vi "single cycle kalman step.vi"(0 "state in":T1, 1 "apply measurement":bool, 2 "z-offset":i16, 5 "location":T4, 9 "pixel values cluster":T3, 11 "feedback channel":enum16{"channel 0", "channel 1", "both"}(ring)=enum."both", 13 "Vz feedback?":bool, 14 "Vxy feedback":bool=TRUE) -> (4 "state out":T1, 8 "kalman counting":bool)   [LabVIEW 2010]
uses:
  kalman 3-axis state.ctl
  integrating single axis kalman state.ctl
  common_typedefs/channels_cluster.ctl
panel:
  # "1 z-level = 3.4*10^-4 * scan amplitude\nat A = 30 um, 1 z-level = 10 nm"
  # "full scan range -> half valid z > 9143 (=143 * 64)"
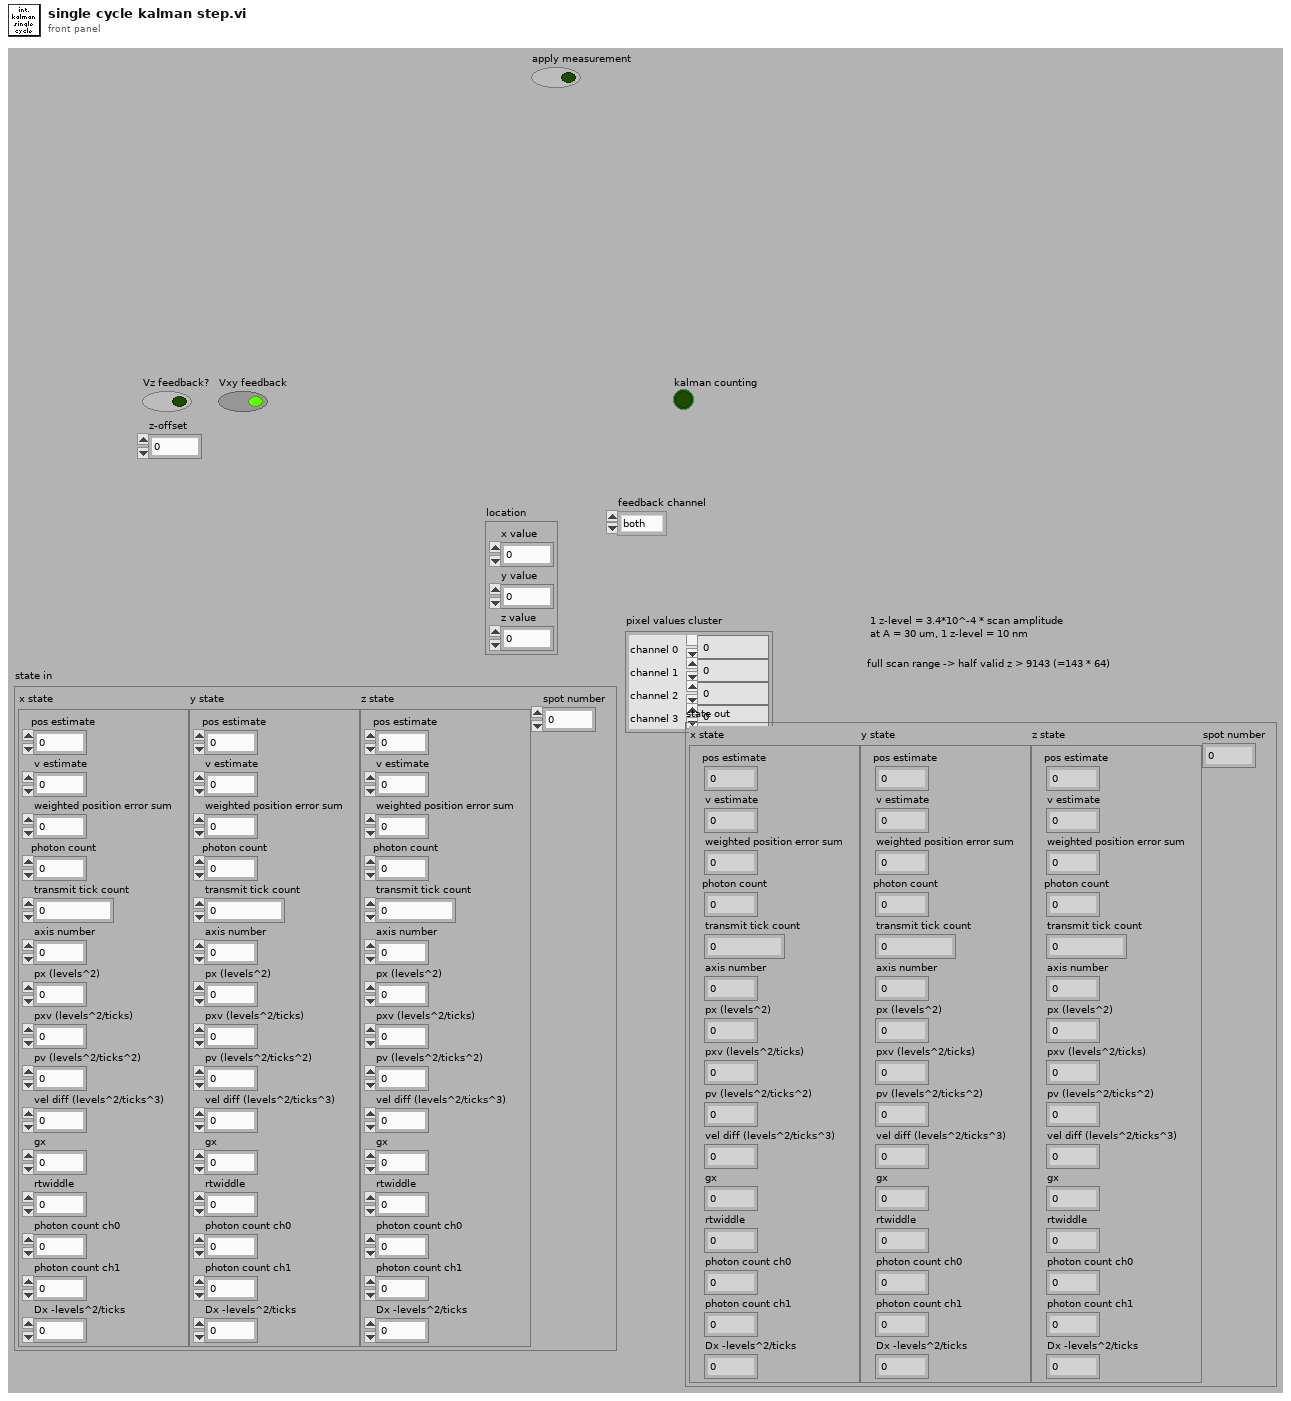
[diagram p1: front panel]
types:
  T1 = typedef "kalman 3-axis state.ctl" = cluster{"x state":T2, "y state":T2, "z state":T2, "spot number":u8}
  T2 = typedef "integrating single axis kalman state.ctl" = cluster{"pos estimate":fxp<+/-,32,16>, "v estimate":fxp<+/-,16,0>, "weighted position error sum":fxp<+/-,32,32>, "photon count":u32, "transmit tick count":u32, "axis number":u8, "px (levels^2)":fxp<+,32,19>, "pxv (levels^2/ticks)":fxp<+,32,2>, "pv (levels^2/ticks^2)":fxp<+,32,-14>, "vel diff (levels^2/ticks^3)":fxp<+,24,-22>, "gx":fxp<+,16,8>, "rtwiddle":fxp<+,16,26>, "photon count ch0":u32, "photon count ch1":u32, "Dx -levels^2/ticks":fxp<+,32,19>}
  T3 = typedef "channels_cluster.ctl" = cluster{"channel 0":u32, "channel 1":u32, "channel 2":u32, "channel 3":u32}
  T4 = cluster{"x value":i16, "y value":i16, "z value":i16}
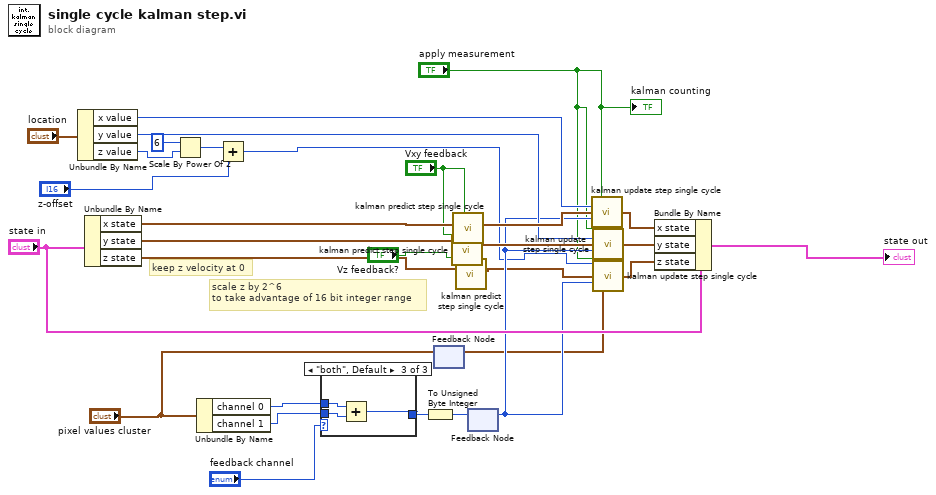
[diagram p0: block diagram]
diagram:
  # "keep z velocity at 0"
  # "scale z by 2^6\nto take advantage of 16 bit integer range"
  n1 = Unbundle By Name("location") -> ("x value"=w28:i16, "y value"=w25:i16, "z value"=w5:i16)
  n2 = Unbundle By Name("state in") -> ("x state"=w30:T2, "y state"=w29:T2, "z state"=w8:T2)
  n3 = Scale By Power Of 2(n=6, x=w5) -> (x*2^n=w4:i16)
  n4 = Unbundle By Name("pixel values cluster") -> ("channel 0"=w19:u32, "channel 1"=w18:u32)
  n5 = Add(x=w4, y="z-offset") -> (x+y=w3:i16)
  n6 = case shown="\"both\", Default" "feedback channel" {
    tunnel: w19 -> [w31 _ w35]
    tunnel: w18 -> [_ w32 w34]
    tunnel: [w31 w32 w33] -> w15
    frame "channel 0" {
    }
    frame "channel 1" {
    }
    frame "both", Default {
      n7 = Add(x=w35, y=w34) -> (x+y=w33:u32)
    }
  }
  n8 = To Unsigned Byte Integer(number=w15) -> (unsigned 8bit integer=w14:u8)
  n9 = feedback-in #1("pixel values cluster") -> ()
  n10 = feedback #1() -> (w9:T3)  [unwired: 1 in]
  n11 = call "kalman predict step single cycle.vi"("v-feedback"="Vxy feedback", "state in"=w29) -> ("state out"=w26:T2)  [unwired: 9 in]
  n12 = call "kalman predict step single cycle.vi"("v-feedback"="Vxy feedback", "state in"=w30) -> ("state out"=w27:T2)  [unwired: 9 in]
  n13 = call "kalman predict step single cycle.vi"("v-feedback"="Vz feedback?", "state in"=w8) -> ("state out"=w11:T2)  [unwired: 9 in]
  n14 = feedback-in #2(w14) -> ()
  n15 = feedback #2() -> (w13:u8)  [unwired: 1 in]
  n16 = call "kalman update step single cycle.vi"("apply measurement?"="apply measurement", "location"=w28, "state in"=w27, "num photons"=w13, "pixel values cluster"=w9) -> ("state out"=w23:T2)  [unwired: 10 in]
  n17 = call "kalman update step single cycle.vi"("apply measurement?"="apply measurement", "location"=w25, "state in"=w26, "num photons"=w13, "pixel values cluster"=w9) -> ("state out"=w22:T2)  [unwired: 10 in]
  n18 = call "kalman update step single cycle.vi"("apply measurement?"="apply measurement", "location"=w3, "state in"=w11, "num photons"=w13, "pixel values cluster"=w9) -> ("state out"=w21:T2)  [unwired: 10 in]
  n19 = Bundle By Name(cluster="state in", "x state"=w23, "y state"=w22, "z state"=w21) -> (→"state out":T1)
  "kalman counting" <- "apply measurement"
